vi "EJERCICIO 10.vi"() -> ()   [LabVIEW 2014]
panel:
  out "Media recortada":dbl
  out "Tercer Cuartil":dbl
  out "Mediana":dbl
  out "Primer Cuartil":dbl
  out "Número Mínimo":dbl
  out "Número Máximo":dbl
  out "Media":dbl
  out "Muestra\nOrdenada":dbl[](array[numeric])
  out "Generacion de\nla muestra":dbl[](array[numeric])
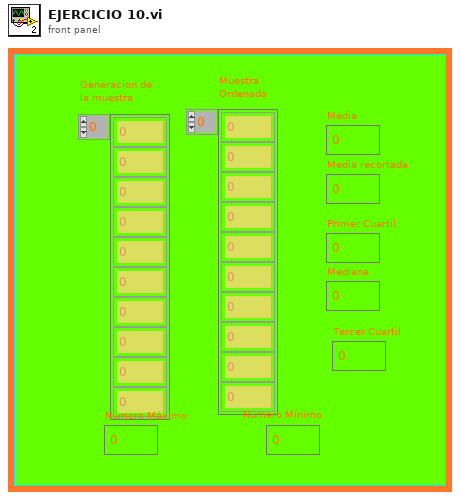
[diagram p1: front panel]
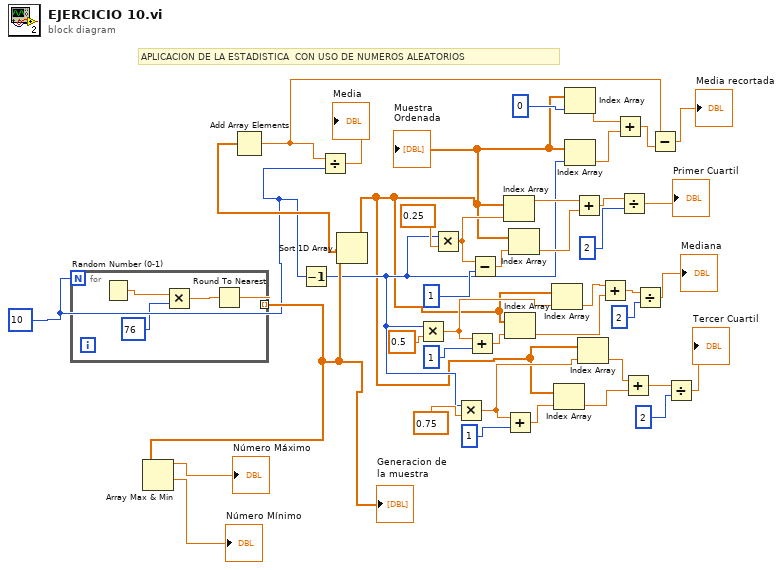
[diagram p0: block diagram]
diagram:
  w8 = 10
  # "APLICACION DE LA ESTADISTICA  CON USO DE NUMEROS ALEATORIOS"
  n1 = for {
    N: w8 -> [_]
    tunnel: [w42] -> w30 mode=indexing
    n2 = Random Number (0-1)() -> (number: 0 to 1=w44:dbl)
    n3 = Multiply(x=w44, y=76) -> (x*y=w43:dbl)
    n4 = Round To Nearest(number=w43) -> (nearest integer value=w42:dbl)
  }
  "Generacion de\nla muestra" <- w30
  n5 = Array Max & Min(array=w30) -> (max value=→"Número Máximo":dbl, min value=→"Número Mínimo":dbl)  [unwired: 2 out]
  n6 = Add Array Elements(numeric array=w30) -> (sum=w9:dbl)
  n7 = Decrement(x=w8) -> (x-1=w5:i32)
  n8 = Divide(x=w9, y=w8) -> (x/y=→"Media":dbl)
  n9 = Sort 1D Array(array=w30) -> (sorted array=w1:dbl[])
  "Muestra\nOrdenada" <- w1
  n10 = Multiply(x=w5, y=0.5) -> (x*y=w23:dbl)
  n11 = Multiply(x=w5, y=0.25) -> (x*y=w33:dbl)
  n12 = Multiply(x=w5, y=0.75) -> (x*y=w2:dbl)
  n13 = Add(x=w23, y=1) -> (x+y=w22:dbl)
  n14 = Subtract(x=w33, y=1) -> (x-y=w31:dbl)
  n15 = Index Array "Index Array"(array=w1, index=w33) -> (element=w29:dbl)
  n16 = Index Array(array=w1, index=w22) -> (element=w4:dbl)
  n17 = Add(x=w2, y=1) -> (x+y=w20:dbl)
  n18 = Index Array(array=w1, index=w31) -> (element=w6:dbl)
  n19 = Index Array(array=w1, index=w23) -> (element=w3:dbl)
  n20 = Index Array(array=w1, index=w20) -> (element=w15:dbl)
  n21 = Index Array(array=w1, index=0) -> (element=w12:dbl)
  n22 = Index Array(array=w1, index=w5) -> (element=w7:dbl)
  n23 = Add(x=w29, y=w6) -> (x+y=w36:dbl)
  n24 = Index Array(array=w1, index=w2) -> (element=w16:dbl)
  n25 = Add(x=w3, y=w4) -> (x+y=w27:dbl)
  n26 = Add(x=w12, y=w7) -> (x+y=w10:dbl)
  n27 = Divide(x=w36, y=2) -> (x/y=→"Primer Cuartil":dbl)
  n28 = Add(x=w16, y=w15) -> (x+y=w18:dbl)
  n29 = Divide(x=w27, y=2) -> (x/y=→"Mediana":dbl)
  n30 = Subtract(x=w9, y=w10) -> (x-y=→"Media recortada":dbl)
  n31 = Divide(x=w18, y=2) -> (x/y=→"Tercer Cuartil":dbl)
